vi "ConfigurePositionController.vi"(0 "axis in":cluster{"keyHandle":u32, "nodeId":u16}={"keyHandle"=0, "nodeId"=1}, 1 "position gains":T2, 2 "feed forward":T1, 3 "error in (no error)":errorcluster) -> (5 "axis out":cluster{"keyHandle":u32, "nodeId":u16}={"keyHandle"=0, "nodeId"=1}, 7 "error out":errorcluster)   [LabVIEW 2019, in "maxonEPOS.lvlib"]
doc: "<B>ConfigurePositionRegulator</B> writes the position regulation gain and the feed forward parameters to the device."
uses:
  Examples/maxonEPOS.lvlib
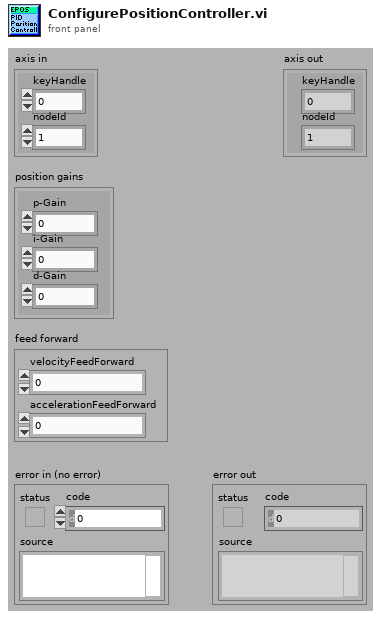
[diagram p1: front panel]
types:
  T1 = cluster{"velocityFeedForward":u64, "accelerationFeedForward":u64}
  T2 = cluster{"p-Gain":u64, "i-Gain":u64, "d-Gain":u64}
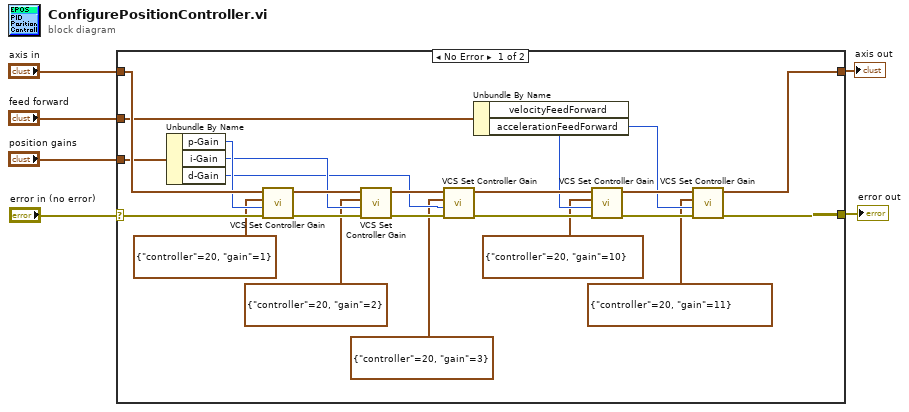
[diagram p0: block diagram]
diagram:
  n1 = case shown="No Error" "error in (no error)" {
    selector: "error in (no error)" -> [w29 w32]
    tunnel: [w30 w32] -> w5
    tunnel: [w23 w31] -> w4
    tunnel: "axis in" -> [w22 w31]
    tunnel: "position gains" -> [w18 _]
    tunnel: "feed forward" -> [w14 _]
    frame No Error {
      n2 = Unbundle By Name(w18) -> ("p-Gain"=w17:u64, "i-Gain"=w16:u64, "d-Gain"=w15:u64)
      n3 = call "VCS Set Controller Gain.vi"("error in (no error)"=w29, "value"=w17, "controller gain"=cluster{"controller":u16, "gain":u16} {"controller"=20, "gain"=1}, "axis in"=w22) -> ("error out"=w28:errorcluster, "axis out"=w21:cluster{"keyHandle":u32, "nodeId":u16})  [unwired: 6 in]
      n4 = call "VCS Set Controller Gain.vi"("error in (no error)"=w28, "value"=w16, "controller gain"=cluster{"controller":u16, "gain":u16} {"controller"=20, "gain"=2}, "axis in"=w21) -> ("error out"=w27:errorcluster, "axis out"=w20:cluster{"keyHandle":u32, "nodeId":u16})  [unwired: 6 in]
      n5 = call "VCS Set Controller Gain.vi"("error in (no error)"=w27, "value"=w15, "controller gain"=cluster{"controller":u16, "gain":u16} {"controller"=20, "gain"=3}, "axis in"=w20) -> ("error out"=w26:errorcluster, "axis out"=w19:cluster{"keyHandle":u32, "nodeId":u16})  [unwired: 6 in]
      n6 = Unbundle By Name(w14) -> ("velocityFeedForward"=w12:u64, "accelerationFeedForward"=w13:u64)
      n7 = call "VCS Set Controller Gain.vi"("error in (no error)"=w26, "value"=w12, "controller gain"=cluster{"controller":u16, "gain":u16} {"controller"=20, "gain"=10}, "axis in"=w19) -> ("error out"=w25:errorcluster, "axis out"=w24:cluster{"keyHandle":u32, "nodeId":u16})  [unwired: 6 in]
      n8 = call "VCS Set Controller Gain.vi"("error in (no error)"=w25, "value"=w13, "controller gain"=cluster{"controller":u16, "gain":u16} {"controller"=20, "gain"=11}, "axis in"=w24) -> ("error out"=w30:errorcluster, "axis out"=w23:cluster{"keyHandle":u32, "nodeId":u16})  [unwired: 6 in]
    }
    frame Error {
    }
  }
  "error out" <- w5
  "axis out" <- w4
